vi "SaveRisRawData.vi"(0 "Filename":string, 1 "Induced Voltage [V]":dbl[][][](array[numeric]), 2 "Volts":dbl[](array[numeric]), 3 "error in (no error)":errorcluster, 4 "SMU Current [nA]":dbl[][][](array[numeric]), 5 "Data formats":string, 8 "Number of data points":i32) -> (10 "error out":errorcluster)   [LabVIEW 2019]
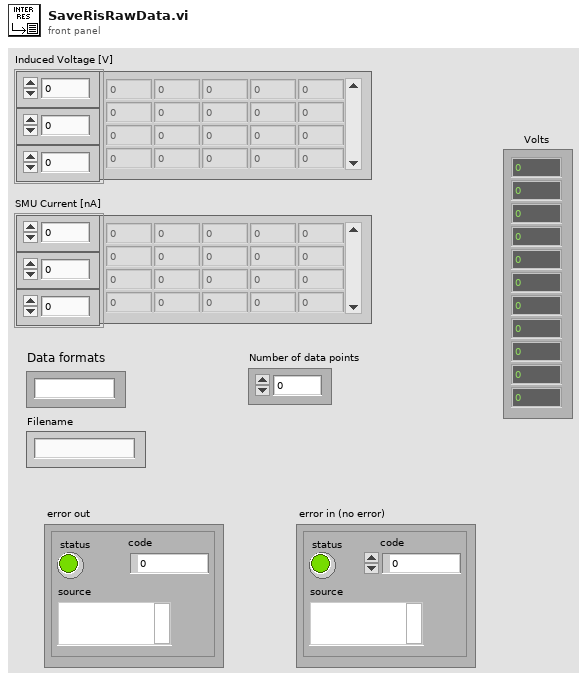
[diagram p1: front panel]
types:
  T1 = enum16{"open", "open or create", "create or replace", "create"}
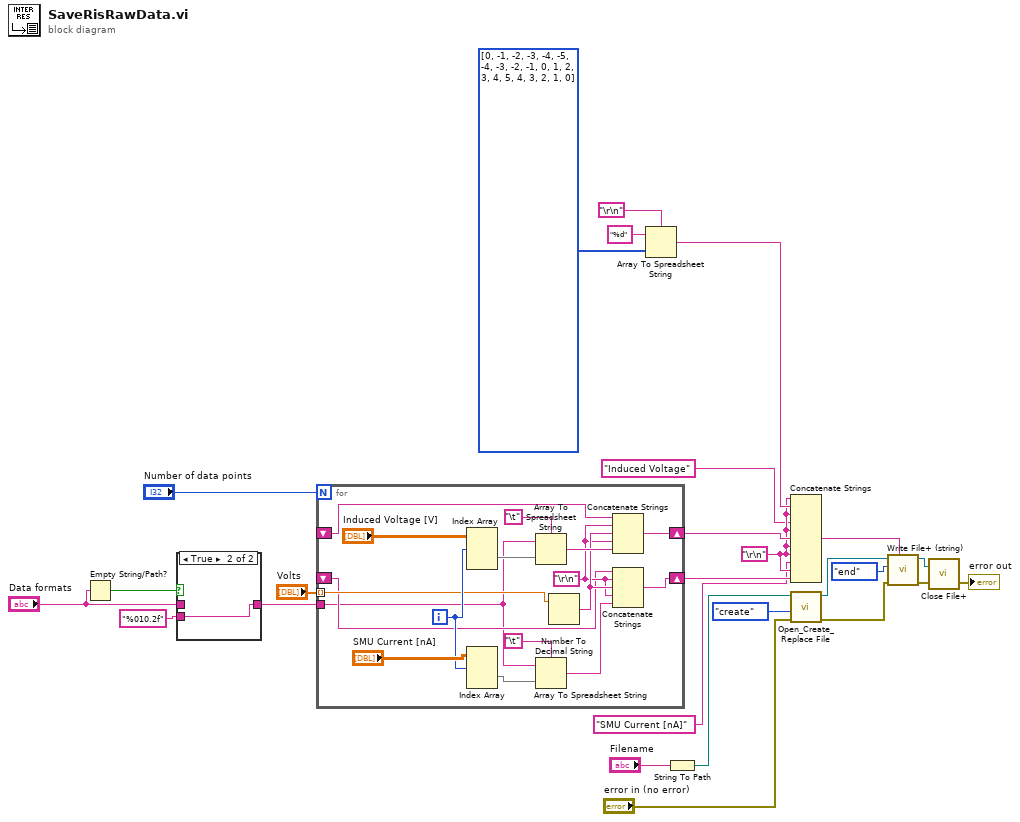
[diagram p0: block diagram]
diagram:
  w19 = "\r\n"
  n1 = Empty String/Path?(string/path="Data formats") -> (empty?=w1:bool)
  n2 = case shown="True" w1 {
    tunnel: "Data formats" -> [w27 _]
    tunnel: [w27 w28] -> w17
    tunnel: "%010.2f" -> [_ w28]
    frame False {
    }
    frame True {
    }
  }
  n3 = for {
    N: "Number of data points" -> [_]
    tunnel: "Volts" -> [w34] mode=indexing
    shift-right: [w37] -> w22
    shift-left: _ -> [w30]
    shift-right: [w35] -> w21
    shift-left: _ -> [w31]
    tunnel: w17 -> [w29]
    i -> [w43]
    w32 = "\r\n"
    n4 = Index Array(array="Induced Voltage [V]", index (dim 0)=w43) -> (element=w40:dbl[][])  [unwired: 2 in]
    n5 = Index Array(array="SMU Current [nA]", index (dim 0)=w43) -> (element=w39:dbl[][])  [unwired: 2 in]
    n6 = Array To Spreadsheet String(delimiter (Tab)="\t", array=w40, 3:w29) -> (spreadsheet string=w38:string)
    n7 = Array To Spreadsheet String(delimiter (Tab)="\t", array=w39, 3:w29) -> (spreadsheet string=w36:string)
    n8 = Number To Decimal String(number=w34) -> (decimal integer string=w33:string)  [unwired: 1 in]
    n9 = Concatenate Strings(w30, w32, w33, w32, w38) -> (w37:string)
    n10 = Concatenate Strings(w31, w32, w33, w32, w36) -> (w35:string)
  }
  n11 = Array To Spreadsheet String(delimiter (Tab)="\r\n", array=i32[] [0, -1, -2, -3, -4, -5, -4, -3, -2, -1, 0, 1, 2, 3, 4, 5, 4, 3, 2, 1, 0] ("Sweep"), 3:"%d" ("format string")) -> (spreadsheet string=w20:string)
  n12 = String To Path(string="Filename") -> (path=w7:path)
  n13 = Concatenate Strings(w19, w20, w19, "Induced Voltage", w19, w22, w19, w19, "SMU Current [nA]", w19, w21) -> (w12:string)
  n14 = call <vilib>:"Open_Create_Replace File.vi"("error in (no error)"="error in (no error)", "function (open:0)"=T1."create", "file path"=w7) -> ("error out"=w4:errorcluster, "refnum"=w3:refnum<file>)  [unwired: 5 in, 2 out]
  n15 = call <vilib>:"Write File+ (string).vi"("string"=w12, "error in (no error)"=w4, "pos mode (rel. to end:1)"=enum16{"start", "end", "current"}."end", "refnum"=w3) -> ("error out"=w14:errorcluster, "dup refnum"=w15:refnum<file>)  [unwired: 3 in, 1 out]
  n16 = call <vilib>:"Close File+.vi"("error in (no error)"=w14, "refnum"=w15) -> ("error out"=→"error out":errorcluster)  [unwired: 3 in, 2 out]
